vi "Set Progress Value.vi"(8 "error in (no error)":errorcluster {"code" format="Error %.0f"}, 10 "Progress Value":i32, 11 "Progress Bar UI In":refnum<class "Progress Bar UI.lvclass">) -> (0 "error out":errorcluster {"code" format="Error %.0f"}, 3 "Progress Bar UI Out":refnum<class "Progress Bar UI.lvclass">)   [LabVIEW 2023, in "Progress Bar UI.lvclass"]
uses:
  Progress Bar UI.lvclass
  Progress Bar UI.lvclass/Progress Bar UI.ctl
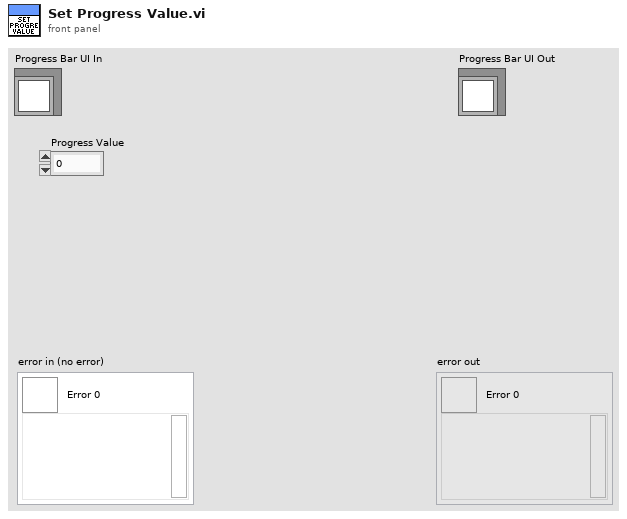
[diagram p1: front panel]
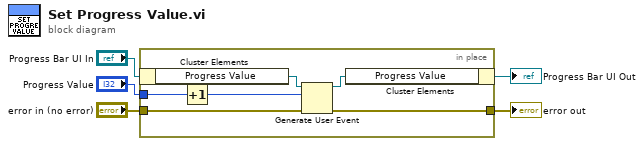
[diagram p0: block diagram]
diagram:
  n1 = in-place {
    in-place-border: "Progress Value" -> [w9]
    in-place-border: "error in (no error)" -> [w8]
    in-place-border: [w7] -> w2
    n2 = in-place-cluster #1("Progress Bar UI In") -> ("Progress Value"=w11:refnum<user-event>)
    n3 = Increment(x=w9) -> (x+1=w6:i32)
    n4 = Generate User Event(user event=w11, event data cluster=w6, error in=w8) -> (user event out=w10:refnum<user-event>, error out=w7:errorcluster)  [unwired: 1 in]
    n5 = in-place-cluster #1("Progress Value"=w10) -> (→"Progress Bar UI Out":refnum<class "Progress Bar UI.lvclass">)
  }
  "error out" <- w2
